vi "test_CCDSetAndGetCleanCount.vi"(6 "Delay between send and receive [ms]":i32=100, 7 "Test should pass":bool=TRUE, 8 "error in":errorcluster, 9 "tear down connection":bool=TRUE, 10 "set-up a connection":bool=TRUE, 11 "device selection":enum16{"monochromator", "CCD", "SCD"}(ring)=enum."CCD") -> (0 "error out":errorcluster)   [LabVIEW 2023]
uses:
  Classes/CCD/CCD.lvclass
  <vilib>/addons/_JKI Toolkits/Caraya/classes/Assert/Assert Equal Value and Type_Variant.vi
  <vilib>/addons/_JKI Toolkits/Caraya/classes/Assert/Assert Not Error.vi
  <vilib>/addons/_JKI Toolkits/Caraya/classes/Test/Test.lvclass
  <vilib>/addons/_JKI Toolkits/Caraya/classes/Assert/Assert.lvclass
panel:
  # "Connector Pane"
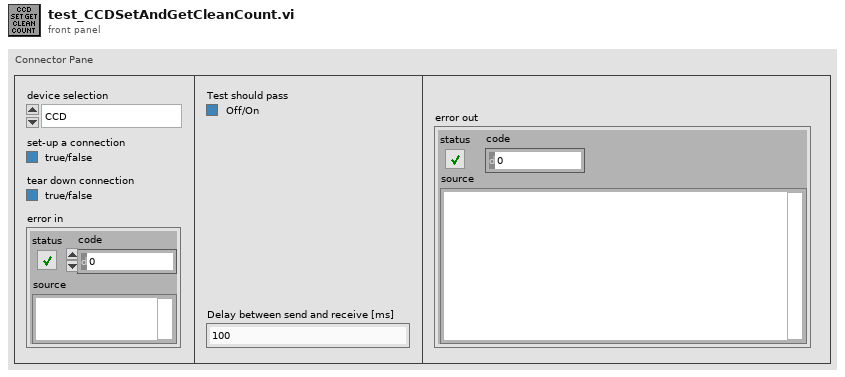
[diagram p1: front panel]
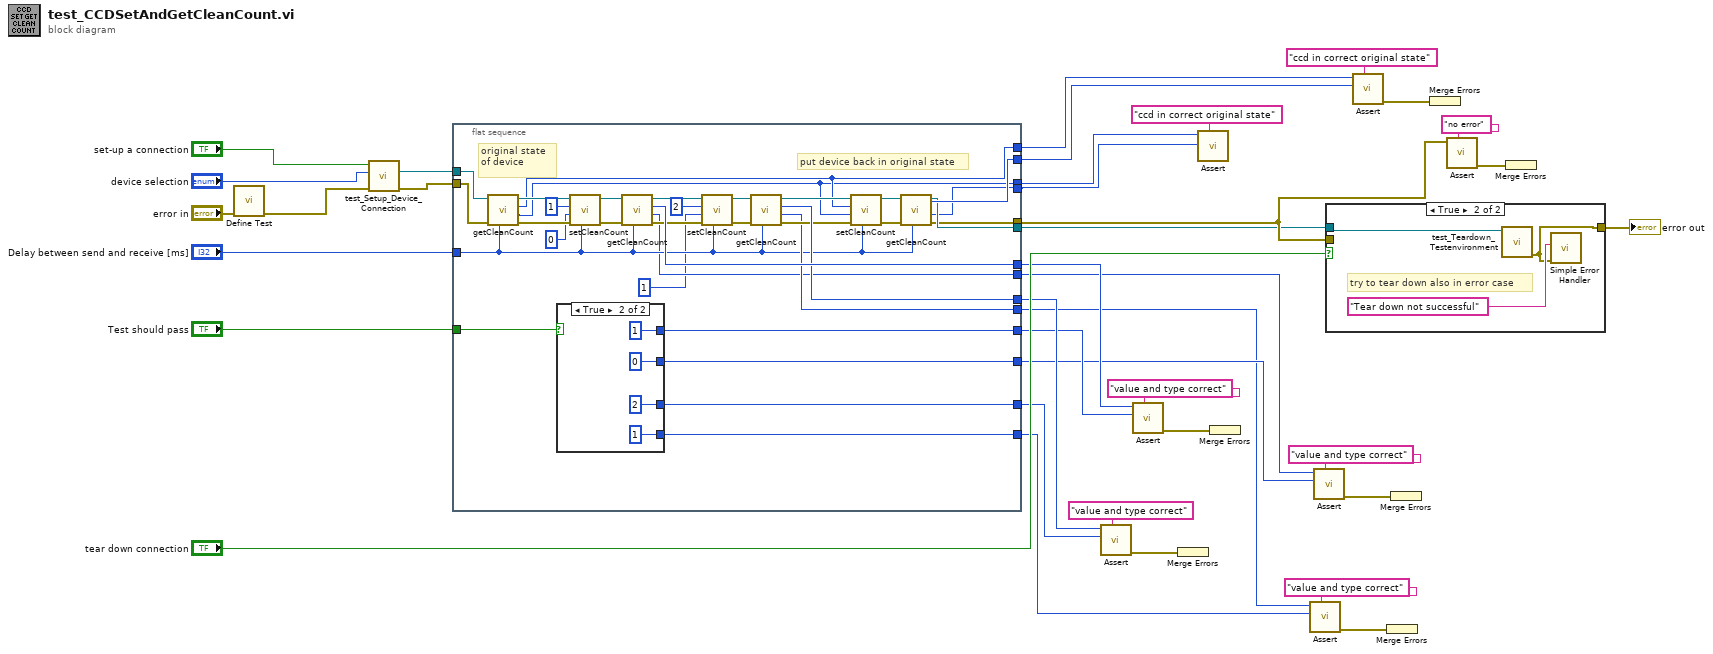
[diagram p0: block diagram]
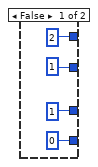
[diagram p2: hidden frame]
diagram:
  n1 = call <vilib>:"Define Test.vi"("error in (no error)"="error in") -> ("error out"=w5:errorcluster)  [unwired: 9 in, 1 out]
  n2 = call "test_Setup_Device_Connection.vi"("error in (no error)"=w5, "device selection"="device selection", "set-up a connection"="set-up a connection") -> ("error out"=w6:errorcluster, "CCD.lvclass"=w4:refnum<class "CCD.lvclass">)  [unwired: 5 in, 2 out]
  n3 = flat-sequence {
    tunnel: w6 -> [w67]
    tunnel: w4 -> [w68]
    tunnel: [w47] -> w28
    tunnel: "Test should pass" -> [w71]
    tunnel: [w48] -> w27
    tunnel: [w55] -> w26
    tunnel: [w70] -> w25
    tunnel: [w61] -> w24
    tunnel: [w69] -> w23
    tunnel: [w50] -> w20
    tunnel: [w49] -> w19
    tunnel: [w46] -> w15
    tunnel: [w40] -> w14
    tunnel: [w45] -> w11
    tunnel: [w44] -> w10
    tunnel: [w43] -> w8
    tunnel: [w42] -> w7
    tunnel: "Delay between send and receive [ms]" -> [w41]
    frame #0 {
      # "put device back in original state"
      # "original state of device"
      n4 = call "getCleanCount.vi"("Delay between send and receive [ms]"=w41, "error in (no error)"=w67, "CCD in"=w68) -> ("error out"=w65:errorcluster, "mode"=w43:i32, "count"=w50:i32, "CCD out"=w66:refnum<class "CCD.lvclass">)  [unwired: 5 in]
      n5 = case shown="True" w71 {
        tunnel: [1 ("exposure time [ms]") 2 ("exposure time [ms]")] -> w70
        tunnel: [2 ("exposure time [ms]") 1 ("exposure time [ms]")] -> w69
        tunnel: [1 ("token") 0 ("token")] -> w46
        tunnel: [0 ("token") 1 ("token")] -> w44
        frame False {
        }
        frame True {
        }
      }
      n6 = call "setCleanCount.vi"("Delay between send and receive [ms]"=w41, "error in (no error)"=w65, "mode"=0 ("token"), "count"=1 ("exposure time [ms]"), "CCD in"=w66) -> ("error out"=w63:errorcluster, "CCD out"=w62:refnum<class "CCD.lvclass">)  [unwired: 3 in, 2 out]
      n7 = call "getCleanCount.vi"("Delay between send and receive [ms]"=w41, "error in (no error)"=w63, "CCD in"=w62) -> ("error out"=w57:errorcluster, "mode"=w40:i32, "count"=w61:i32, "CCD out"=w58:refnum<class "CCD.lvclass">)  [unwired: 5 in]
      n8 = call "setCleanCount.vi"("Delay between send and receive [ms]"=w41, "error in (no error)"=w57, "mode"=1 ("token"), "count"=2 ("exposure time [ms]"), "CCD in"=w58) -> ("error out"=w60:errorcluster, "CCD out"=w59:refnum<class "CCD.lvclass">)  [unwired: 3 in, 2 out]
      n9 = call "getCleanCount.vi"("Delay between send and receive [ms]"=w41, "error in (no error)"=w60, "CCD in"=w59) -> ("error out"=w52:errorcluster, "mode"=w45:i32, "count"=w55:i32, "CCD out"=w53:refnum<class "CCD.lvclass">)  [unwired: 5 in]
      n10 = call "setCleanCount.vi"("Delay between send and receive [ms]"=w41, "error in (no error)"=w52, "mode"=w43, "count"=w50, "CCD in"=w53) -> ("error out"=w54:errorcluster, "CCD out"=w51:refnum<class "CCD.lvclass">)  [unwired: 3 in, 2 out]
      n11 = call "getCleanCount.vi"("Delay between send and receive [ms]"=w41, "error in (no error)"=w54, "CCD in"=w51) -> ("error out"=w47:errorcluster, "mode"=w42:i32, "count"=w49:i32, "CCD out"=w48:refnum<class "CCD.lvclass">)  [unwired: 5 in]
    }
  }
  n12 = call-poly <vilib>:"Assert.vi"("Label"="value and type correct" ("Label (VI Title)"), "Y"=w25, "X"=w26) -> ("error out"=w36:errorcluster)  [unwired: 7 in, 1 out]
  n13 = call-poly <vilib>:"Assert.vi"("Label"="value and type correct" ("Label (VI Title)"), "Y"=w23, "X"=w24) -> ("error out"=w35:errorcluster)  [unwired: 7 in, 1 out]
  n14 = Merge Errors(w36) -> ()  [unwired: 1 out]
  n15 = call-poly <vilib>:"Assert.vi"("Label"="ccd in correct original state" ("Label (VI Title)"), "Y"=w7, "X"=w8) -> ()  [unwired: 7 in, 2 out]
  n16 = Merge Errors(w35) -> ()  [unwired: 1 out]
  n17 = call-poly <vilib>:"Assert.vi"("Label"="value and type correct" ("Label (VI Title)"), "Y"=w10, "X"=w11) -> ("error out"=w13:errorcluster)  [unwired: 7 in, 1 out]
  n18 = call-poly <vilib>:"Assert.vi"("Label"="value and type correct" ("Label (VI Title)"), "Y"=w15, "X"=w14) -> ("error out"=w16:errorcluster)  [unwired: 7 in, 1 out]
  n19 = case shown="True" "tear down connection" {
    tunnel: w27 -> [_ w82]
    tunnel: [w80 w81] -> w18
    tunnel: w28 -> [w80 _]
    frame False {
    }
    frame True {
      # "try to tear down also in error case"
      n20 = call "test_Teardown_Testenvironment.vi"("GenericDevice.lvclass"=w82) -> ("error out"=w81:errorcluster)  [unwired: 9 in, 1 out]
      n21 = call <vilib>:"Simple Error Handler.vi"("error source (\" \")"="Tear down not successful" ("error source (\" \")"), "error in (no error)"=w81) -> ()  [unwired: 3 in, 5 out]
    }
  }
  "error out" <- w18
  n22 = call-poly <vilib>:"Assert.vi"("Label"="ccd in correct original state" ("Label (VI Title)"), "Y"=w19, "X"=w20) -> ("error out"=w22:errorcluster)  [unwired: 7 in, 1 out]
  n23 = Merge Errors(w13) -> ()  [unwired: 1 out]
  n24 = Merge Errors(w16) -> ()  [unwired: 1 out]
  n25 = Merge Errors(w22) -> ()  [unwired: 1 out]
  n26 = call-poly <vilib>:"Assert.vi"("Label"="no error" ("Label (VI Title)"), "Not Error?"=w28) -> ("error out"=w30:errorcluster)  [unwired: 8 in, 1 out]
  n27 = Merge Errors(w30) -> ()  [unwired: 1 out]
